vi "Set New Status.vi"(8 "error in (no error)":errorcluster, 10 "Status":T1, 11 "abs_Parallel in":refnum<class "abs_Parallel.lvclass">) -> (0 "error out":errorcluster, 3 "abs_Parallel out":refnum<class "abs_Parallel.lvclass">)   [LabVIEW 2021, in "BT.lvlib" / "abs_Parallel.lvclass"]
uses:
  abs_Parallel.lvclass
  C:/Users/Tim/Documents/LabVIEW/2021/Behaviour Tree/Source/abs_Composite/abs_Composite.lvclass
  abs_Node/Status.ctl
  abs_Composite/abs_Composite.lvclass/abs_Composite.ctl
  abs_Parallel.lvclass/abs_Parallel.ctl
  abs_Composite/Properties/Read Index.vi
  abs_Node/abs_Node.lvclass
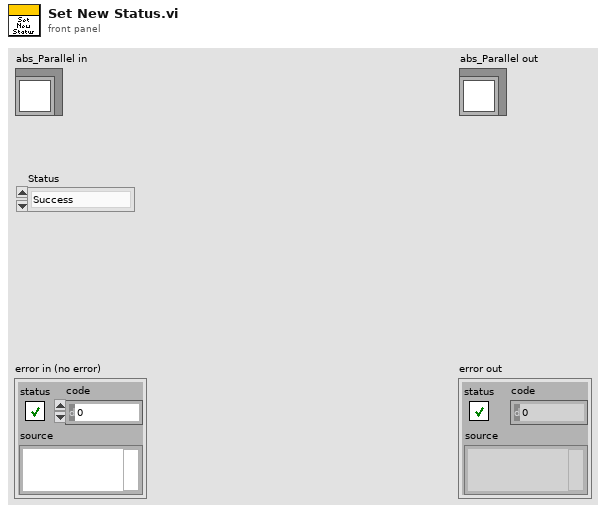
[diagram p1: front panel]
types:
  T1 = typedef "BT.lvlib/abs_Node.lvclass/Status.ctl" = enum16{"Success", "Failure", "Running"}
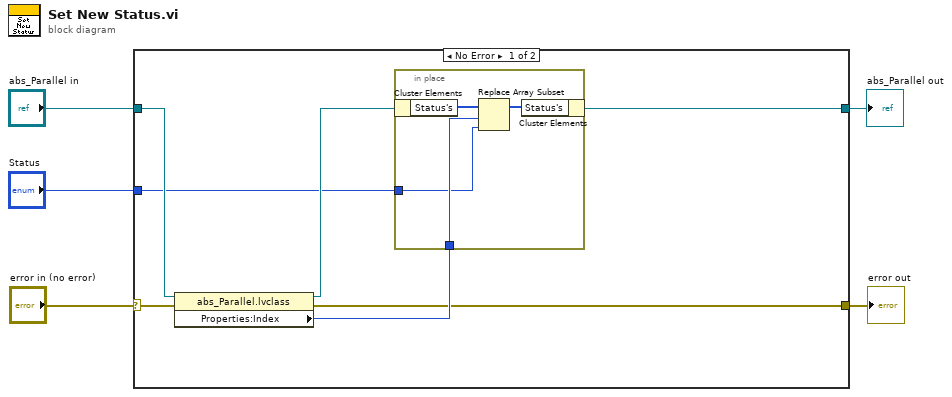
[diagram p0: block diagram]
diagram:
  n1 = case shown="No Error" "error in (no error)" {
    selector: "error in (no error)" -> [w12 w18]
    tunnel: [w7 w18] -> w4
    tunnel: [w8 w17] -> w2
    tunnel: "abs_Parallel in" -> [w11 w17]
    tunnel: "Status" -> [w6 _]
    frame No Error {
      n2 = property class="abs_Parallel.lvclass"(reference=w11, error in=w12) -> (reference out=w10:refnum<class "abs_Parallel.lvclass">, error out=w7:errorcluster, "Properties:Index"=w9:i32)
      n3 = in-place {
        in-place-border: w9 -> [w15]
        in-place-border: w6 -> [w13]
        n4 = in-place-cluster #1(w10) -> ("Status's"=w16:T1[])
        n5 = Replace Array Subset(array=w16, new element=w13, index=w15) -> (w14:T1[])
        n6 = in-place-cluster #1("Status's"=w14) -> (w8:refnum<class "abs_Parallel.lvclass">)
      }
    }
    frame Error {
    }
  }
  "error out" <- w4
  "abs_Parallel out" <- w2
